vi "svx_Colormap Resize Pane for Scale and Cursor Legend.vi"(10 "Color Map in":refnum<vi>, 11 "Container ref":refnum<vi>) -> ()   [LabVIEW 2017, in "SVX Colormap.xctl"]
uses:
  <vilib>/addons/_XControls/Colormap/SVX Colormap.xctl
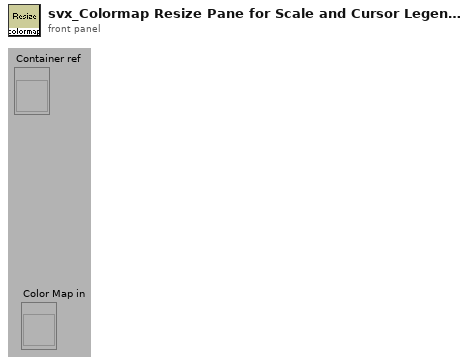
[diagram p1: front panel]
types:
  T1 = typedef "LVRectTypeDef.ctl" = cluster{"Left":i16, "Top":i16, "Right":i16, "Bottom":i16}
  T2 = typedef "LVBoundsTypeDef.ctl" = cluster{"Width":u32, "Height":u32}
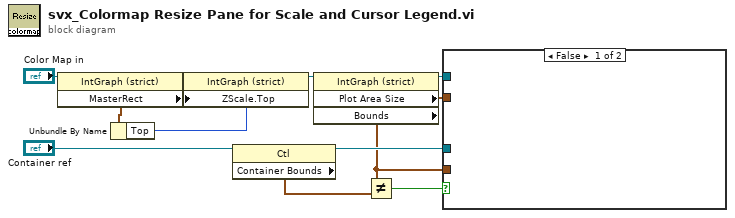
[diagram p0: block diagram]
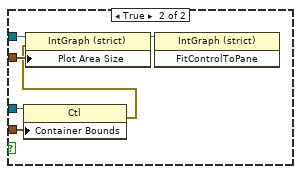
[diagram p2: hidden frame]
diagram:
  n1 = property class="IntGraph (strict)"(reference="Color Map in") -> (reference out=w1:refnum<vi>, "MasterRect"=w3:T1)  [unwired: 1 in, 1 out]
  n2 = Unbundle By Name(w3) -> ("Top"=w2:i16)
  n3 = property class="IntGraph (strict)"(reference=w1, "ZScale.Top"=w2) -> (reference out=w10:refnum<vi>)  [unwired: 1 in, 1 out]
  n4 = property class="Ctl"(reference="Container ref") -> (reference out=w7:refnum<vi>, "Container Bounds"=w6:T2)  [unwired: 1 in, 1 out]
  n5 = property class="IntGraph (strict)"(reference=w10) -> (reference out=w11:refnum<vi>, "Plot Area Size"=w9:T2, "Bounds"=w4:T2)  [unwired: 1 in, 1 out]
  n6 = Not Equal?(x=w4, y=w6) -> (x != y?=w5:bool)
  n7 = case shown="False" w5 {
    tunnel: w11 -> [_ w18]
    tunnel: w9 -> [_ w16]
    tunnel: w7 -> [_ w15]
    tunnel: w4 -> [_ w14]
    frame False {
    }
    frame True {
      n8 = property class="Ctl"(reference=w15, "Container Bounds"=w14) -> (error out=w13:errorcluster)  [unwired: 1 in, 1 out]
      n9 = property class="IntGraph (strict)"(reference=w18, error in=w13, "Plot Area Size"=w16) -> (reference out=w17:refnum<vi>)  [unwired: 1 out]
      n10 = invoke class="IntGraph (strict)" method="FitControlToPane"(reference=w17) -> ()  [unwired: 2 in, 3 out]
    }
  }
